vi "Go To Fine Axis Position (um).vi"(8 "error in":errorcluster, 10 "Fine Axis Position (um)":dbl[unit], 11 "GPIB # (in): def. 6":string="6") -> (0 "error out":errorcluster, 3 "GPIB # (out)":string="6")   [LabVIEW 2017]
uses:
  mc2mc4.llb/MC2/MC4 Wait&ParseSRQ.vi
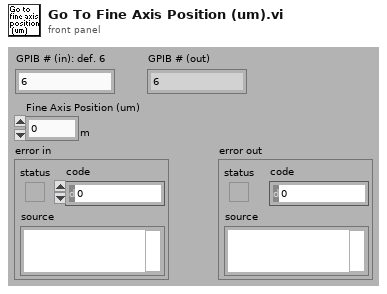
[diagram p1: front panel]
types:
  T1 = enum16{"fine axis move complete", "coarse axis move complete", "either axis move complete", "an axis has reached travel limit"}
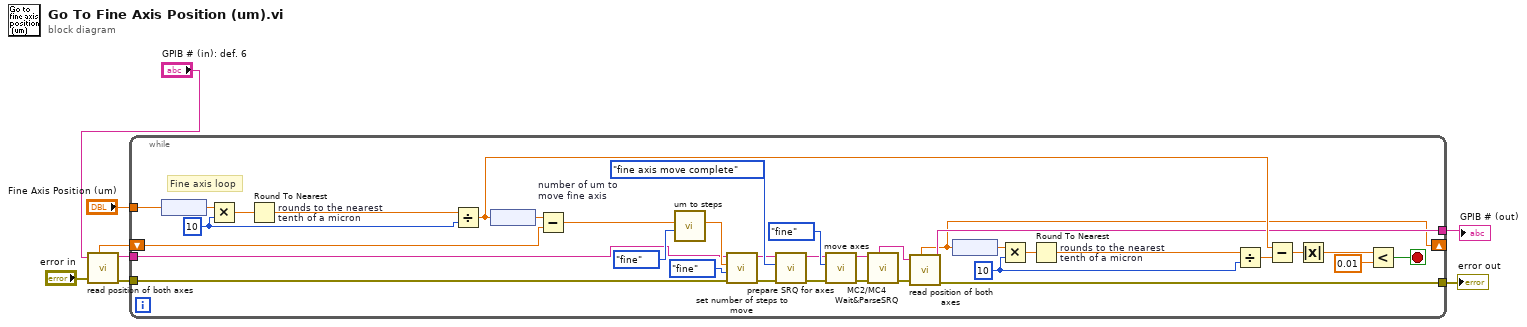
[diagram p0: block diagram]
diagram:
  n1 = call "read position of both axes.vi"("GPIB # (in): def. 6"="GPIB # (in): def. 6", "error in (no error)"="error in") -> ("fine axis (um)"=w4:ext[unit], "GPIB # (out)"=w2:string, "error out"=w7:errorcluster)  [unwired: 6 out]
  n2 = while {
    tunnel: "Fine Axis Position (um)" -> [w27]
    tunnel: w7 -> [w39]
    tunnel: [w38] -> w8
    shift-right: [w9] -> _
    shift-left: w4 -> [w37]
    tunnel: w2 -> [w15]
    tunnel: [w10] -> w1
    stop <- w16 stop-if-true
    w24 = i8 10 ("y")
    w31 = i8 10 ("y")
    # "Fine axis loop"
    n3 = node(w27) -> (w28:dbl)
    n4 = Multiply(x=w28, y=w31) -> (x*y=w29:dbl)
    n5 = Round To Nearest "rounds to the nearest tenth of a micron"(number=w29) -> (nearest integer value=w30:dbl)
    n6 = Divide(x=w30, y=w31) -> (x/y=w25:dbl)
    n7 = node(w25) -> (w26:dbl[unit])
    n8 = Subtract "number of um to\nmove fine axis"(x=w26, y=w37) -> (x-y=w43:ext[unit])
    n9 = call "um to steps.vi"("axis (default = fine)"=enum16{"fine", "coarse"}."fine", "position (microns)"=w43) -> ("steps"=w42:dbl)  [unwired: 9 out]
    n10 = call "set number of steps to move.vi"("error in"=w39, "axis (def: fine)"=enum16{"fine", "coarse"}."fine", "number of steps to set"=w42, "GPIB # (in): def. 6"=w15) -> ("error out"=w36:errorcluster, "GPIB # (out)"=w14:string)  [unwired: 6 out]
    n11 = call "prepare SRQ for axes.vi"("error in (no error)"=w36, "category"=T1."fine axis move complete", "GPIB # (in): def. 6"=w14) -> ("error out"=w35:errorcluster, "GPIB # (out):"=w13:string)  [unwired: 7 out]
    n12 = call "move axes.vi"("error in"=w35, "stage to move"=enum16{"both", "fine", "coarse"}."fine", "GPIB # (in): def. 6"=w13) -> ("error out"=w34:errorcluster, "GPIB # (out)"=w12:string)  [unwired: 7 out]
    n13 = call "MC2/MC4 Wait&ParseSRQ.vi"("error in (no error)"=w34, "GPIB # (in): def. 6"=w12) -> ("error out"=w33:errorcluster, "GPIB #(out): def. 6"=w11:string)  [unwired: 8 out]
    n14 = call "read position of both axes.vi"("GPIB # (in): def. 6"=w11, "error in (no error)"=w33) -> ("fine axis (um)"=w9:ext[unit], "GPIB # (out)"=w10:string, "error out"=w38:errorcluster)  [unwired: 6 out]
    n15 = node(w9) -> (w21:ext)
    n16 = Multiply(x=w21, y=w24) -> (x*y=w22:ext)
    n17 = Round To Nearest "rounds to the nearest tenth of a micron"(number=w22) -> (nearest integer value=w23:ext)
    n18 = Divide(x=w23, y=w24) -> (x/y=w20:ext)
    n19 = Subtract(x=w25, y=w20) -> (x-y=w17:ext)
    n20 = Absolute Value(x=w17) -> (abs(x)=w19:ext)
    n21 = Less?(x=w19, y=0.01) -> (x < y?=w16:bool)
  }
  "error out" <- w8
  "GPIB # (out)" <- w1
